vi "GetObjectConfiguration.vi"(8 "error in (no error)":errorcluster, 11 "SMO":refnum<class "SMO.lvclass">) -> (0 "error out":errorcluster, 1 "Values":variant[](array[variant]), 2 "Keys":string[](array[string]), 3 "SMO out":refnum<class "SMO.lvclass">)   [LabVIEW 2013, in "SMO.lvclass"]
uses:
  SMO.lvclass
  Support/Attribute.Config/Attribute.Config.lvclass
panel:
  # "For instructions on how to use the JKI State Machine Objects, examples and video tutorials, visit:\nhttp://jki.net/state-machine-objects/\n\nJKI State Machine Objects™\nhttp://jki.net/state-machine-objects/\nCopyright (C) 2005-2015, JKI <info@jki.net>\nALL RIGHTS RESERVED"
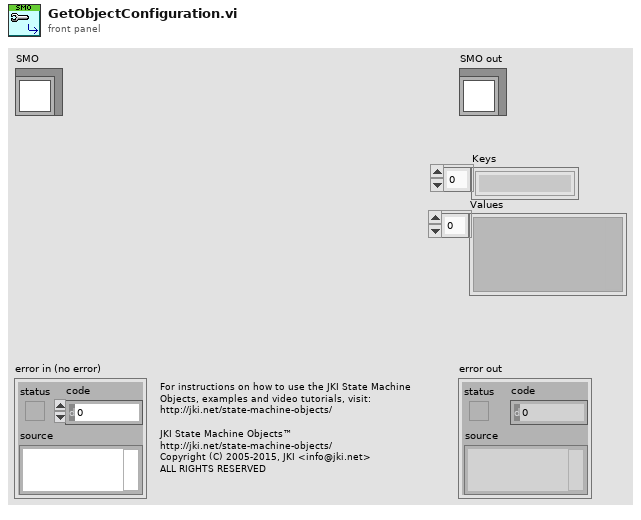
[diagram p1: front panel]
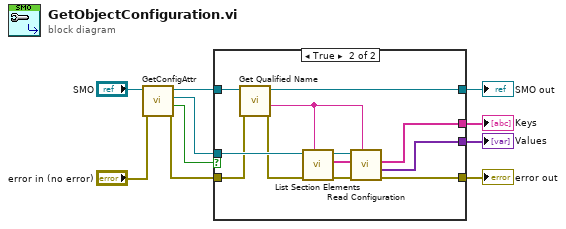
[diagram p0: block diagram]
diagram:
  n1 = call "GetConfigAttr.vi"("error in (no error)"="error in (no error)", "SMO in"="SMO") -> ("error out"=w3:errorcluster, "found"=w6:bool, "Attribute.Config"=w5:refnum<class "Attribute.Config.lvclass">, "SMO out"=w7:refnum<class "SMO.lvclass">)  [unwired: 6 in]
  n2 = case shown="True" w6 {
    tunnel: w5 -> [_ w22]
    tunnel: w7 -> [w12 w17]
    tunnel: [w12 w13] -> w10
    tunnel: w3 -> [w11 w16]
    tunnel: [w11 w24] -> w9
    tunnel: [_ w19] -> w2
    tunnel: [_ w18] -> w1
    frame False {
    }
    frame True {
      n3 = call "Get Qualified Name.vi"("error in (no error)"=w16, "SMO"=w17) -> ("error out"=w15:errorcluster, "Reserved Qualified Name"=w14:string, "SMO out"=w13:refnum<class "SMO.lvclass">)  [unwired: 6 in, 1 out]
      n4 = call-dynamic "List Section Elements.vi"("Qualified Name"=w14, "error in (no error)"=w15, "Attribute.Config in"=w22) -> ("error out"=w23:errorcluster, "Keys"=w20:string[], "Attribute.Config out"=w21:refnum<class "Attribute.Config.lvclass">)  [unwired: 6 in]
      n5 = call-dynamic "Read Configuration.vi"("Qualified Name"=w14, "error in (no error)"=w23, "URIs"=w20, "Attribute.Config in"=w21) -> ("error out"=w24:errorcluster, "Values"=w18:variant[], "URIs dup"=w19:string[])  [unwired: 4 in, 1 out]
    }
  }
  "error out" <- w9
  "SMO out" <- w10
  "Keys" <- w2
  "Values" <- w1
